vi "程序框图存储为PNG.vi"() -> ()   [LabVIEW 2011]
panel:
  in  "仅可见区域":bool
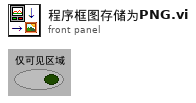
[diagram p1: front panel]
types:
  T1 = typedef "imagedata.ctl" = cluster{"image type":i32, "image depth":i32, "image":u8[], "mask":u8[], "colors":u32[], "Rectangle":cluster{"left":i16, "top":i16, "right":i16, "bottom":i16}}
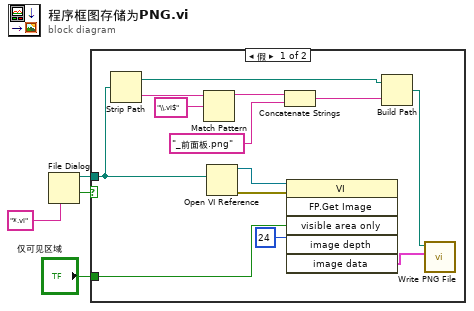
[diagram p0: block diagram]
diagram:
  n1 = File Dialog(6:"*.vi" ("default name")) -> (1:w2:bool, 3:w3:path)  [unwired: 6 in, 2 out]
  n2 = case shown="假" w2 {
    tunnel: w3 -> [w14 _]
    tunnel: "仅可见区域" -> [w6 _]
    frame False {
      n3 = Strip Path(path=w14) -> (stripped path=w12:path, name=w13:string)
      n4 = Match Pattern(string=w13, regular expression="\\.vi$") -> (before substring=w11:string)  [unwired: 1 in, 3 out]
      n5 = Open VI Reference(vi path=w14) -> (vi reference=w17:refnum<vi>, error out=w7:errorcluster)  [unwired: 5 in]
      n6 = Concatenate Strings(w11, "_前面板.png" ("string")) -> (w9:string)
      n7 = invoke class="VI" method="FP.Get Image"(reference=w17, error in=w7, "visible area only"=w6, "image depth"=24) -> ("image data"=w5:T1)  [unwired: 2 in, 5 out]
      n8 = Build Path(base path=w12, name or relative path=w9) -> (appended path=w8:path)
      n9 = call <vilib>:"Write PNG File.vi"("image data"=w5, "path to PNG file"=w8) -> ()  [unwired: 8 in, 2 out]
    }
    frame True {
    }
  }
